vi "Adapt FP.vi"(8 "error in":errorcluster, 11 "ref":refnum<vi>) -> (0 "error out":errorcluster)   [LabVIEW 2009, in "POLARIS Vision utility.lvlib"]
uses:
  POLARIS Vision utility.lvlib
  control position.ctl
  <vilib>/Utility/miscctls.llb/LVPositionTypeDef.ctl
  <vilib>/Utility/miscctls.llb/LVBoundsTypeDef.ctl
  <vilib>/Utility/xml.llb/Write to XML File(string).vi
panel:
  in  "thin":bool
  in  "thick":bool
  in  "wide":bool
  in  "narroq":bool
  in  "bottom":bool
  in  "Top":bool
  in  "Right":bool
  in  "Left":bool
  in  "stop":bool
  in  "Select Element":u16(ring) items=["Numeric", "String", "String 2", "stop", "Path"]
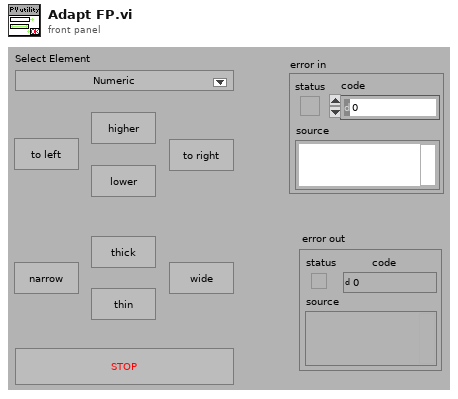
[diagram p1: front panel]
types:
  T1 = typedef "control position.ctl" = cluster{"ControlName":string, "Position":T2, "Size":T3}
  T2 = typedef "LVPositionTypeDef.ctl" = cluster{"Left":i32, "Top":i32}
  T3 = typedef "LVBoundsTypeDef.ctl" = cluster{"Width":u32, "Height":u32}
  T4 = enum32{"invalid app kind", "Development System", "Run Time System", "Student Edition", "Embedded LabVIEW", "Evaluation", "Custom"}
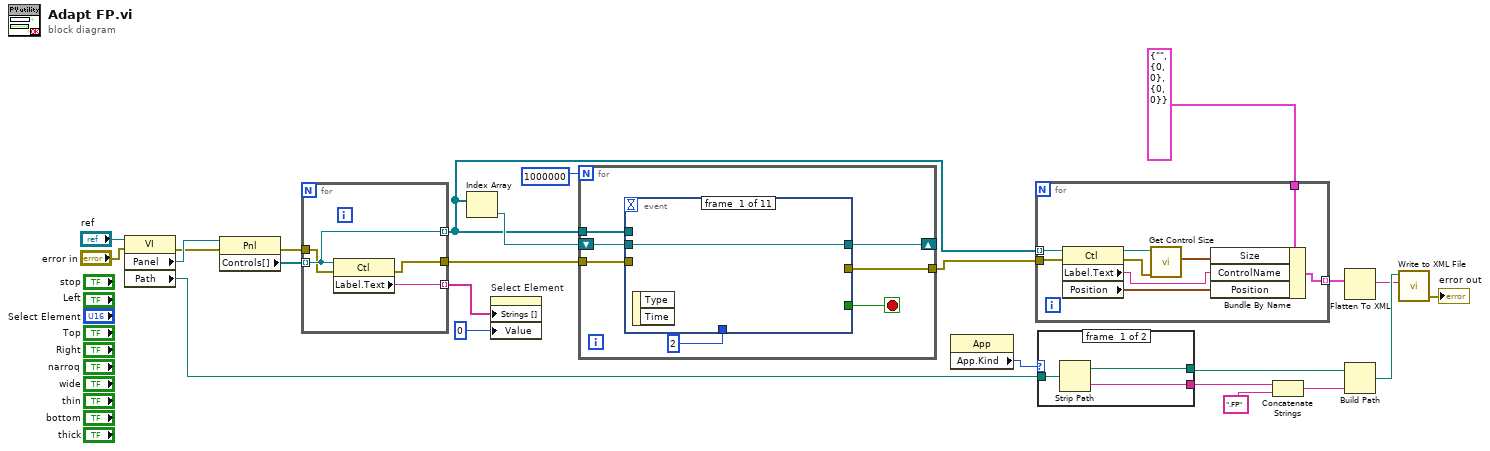
[diagram p0: block diagram]
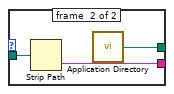
[diagram p2: hidden frame]
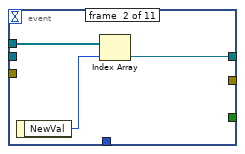
[diagram p3: hidden frame]
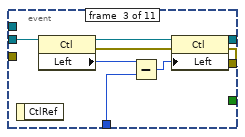
[diagram p4: hidden frame]
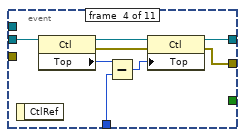
[diagram p5: hidden frame]
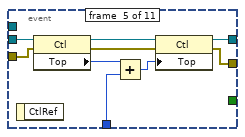
[diagram p6: hidden frame]
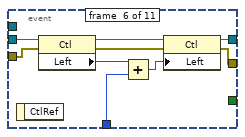
[diagram p7: hidden frame]
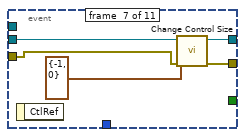
[diagram p8: hidden frame]
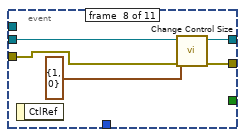
[diagram p9: hidden frame]
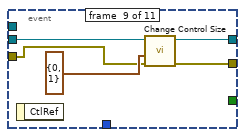
[diagram p10: hidden frame]
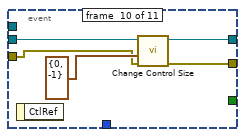
[diagram p11: hidden frame]
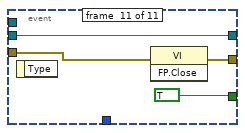
[diagram p12: hidden frame]
diagram:
  n1 = property class="VI"(reference="ref", error in="error in") -> (error out=w22:errorcluster, "Panel"=w23:refnum<vi>, "Path"=w17:path)  [unwired: 1 out]
  n2 = property class="Pnl"(reference=w23, error in=w22) -> (error out=w6:errorcluster, "Controls[]"=w21:refnum<vi>[])  [unwired: 1 out]
  n3 = for {
    tunnel: w21 -> [w27] mode=indexing
    tunnel: [w28] -> w20 mode=indexing
    tunnel: [w27] -> w1 mode=indexing
    tunnel: w6 -> [w26]
    tunnel: [w25] -> w5
    n4 = property class="Ctl"(reference=w27, error in=w26) -> (error out=w25:errorcluster, "Label.Text"=w28:string)  [unwired: 1 out]
  }
  n5 = Index Array(array=w1) -> (element=w19:refnum<vi>)  [unwired: 1 in]
  n6 = property on="Select Element" class="Ring (strict)"("Strings []"=w20, "Value"=u16 0 ("Select Element")) -> ()  [unwired: 2 in, 2 out]
  n7 = for {
    N: 1000000 -> [_]
    tunnel: w1 -> [w35]
    shift-right: [w31] -> _
    shift-left: w19 -> [w34]
    tunnel: [w33] -> w4
    tunnel: w5 -> [w30]
    stop <- w32 stop-if-true
    n8 = event shown="[10] \"stop\": Value Change" {
      selector: _ -> [_ _ _ _ _ _ _ _ _ _ _]
      dyn-events: _ -> [_ _ _ _ _ _ _ _ _ _ _]
      timeout: _ -> [_ _ _ _ _ _ _ _ _ _ _]
      tunnel: w35 -> [_ w39 _ _ _ _ _ _ _ _ _]
      tunnel: [_ _ _ _ _ _ _ _ _ _ TRUE] -> w32
      tunnel: [w36 w38 w43 w51 w60 w69 w78 w83 w88 w93 w96] -> w31
      tunnel: w34 -> [w36 _ w44 w52 w61 w73 w77 w82 w87 w92 w96]
      tunnel: [_ _ w42 w49 w58 w67 w75 w80 w85 w90 w95] -> w33
      tunnel: w30 -> [_ _ _ _ w57 w66 w74 w79 w84 w89 w94]
      tunnel: 2 ("y") -> [_ _ w40 w48 w56 w65 _ _ _ _ _]
      event #0 {
        n9 = event-data() -> ()  [unwired: 1 in, 2 out]
      }
      event #1 {
        n10 = event-data() -> ("NewVal"=w37:u16)  [unwired: 1 in]
        n11 = Index Array(array=w39, index=w37) -> (element=w38:refnum<vi>)
      }
      event #2 {
        n12 = event-data() -> ()  [unwired: 1 in, 1 out]
        n13 = property class="Ctl"(reference=w44) -> (reference out=w45:refnum<vi>, error out=w41:errorcluster, "Left"=w47:i32)  [unwired: 1 in]
        n14 = Subtract(x=w47, y=w40) -> (x-y=w46:i32)
        n15 = property class="Ctl"(reference=w45, error in=w41, "Left"=w46) -> (reference out=w43:refnum<vi>, error out=w42:errorcluster)
      }
      event #3 {
        n16 = event-data() -> ()  [unwired: 1 in, 1 out]
        n17 = property class="Ctl"(reference=w52) -> (reference out=w53:refnum<vi>, error out=w50:errorcluster, "Top"=w55:i32)  [unwired: 1 in]
        n18 = Subtract(x=w55, y=w48) -> (x-y=w54:i32)
        n19 = property class="Ctl"(reference=w53, error in=w50, "Top"=w54) -> (reference out=w51:refnum<vi>, error out=w49:errorcluster)
      }
      event #4 {
        n20 = event-data() -> ()  [unwired: 1 in, 1 out]
        n21 = property class="Ctl"(reference=w61, error in=w57) -> (reference out=w62:refnum<vi>, error out=w59:errorcluster, "Top"=w64:i32)
        n22 = Add(x=w64, y=w56) -> (x+y=w63:i32)
        n23 = property class="Ctl"(reference=w62, error in=w59, "Top"=w63) -> (reference out=w60:refnum<vi>, error out=w58:errorcluster)
      }
      event #5 {
        n24 = event-data() -> ()  [unwired: 1 in, 1 out]
        n25 = property class="Ctl"(reference=w73, error in=w66) -> (reference out=w70:refnum<vi>, error out=w68:errorcluster, "Left"=w72:i32)
        n26 = Add(x=w72, y=w65) -> (x+y=w71:i32)
        n27 = property class="Ctl"(reference=w70, error in=w68, "Left"=w71) -> (reference out=w69:refnum<vi>, error out=w67:errorcluster)
      }
      event #6 {
        n28 = event-data() -> ()  [unwired: 1 in, 1 out]
        n29 = call "Change Control Size.vi"("error in (no error)"=w74, "dSize"=cluster{"Width":i32, "Height":i32} {"Width"=-1, "Height"=0}, "Ctl Refnum"=w77) -> ("error out"=w75:errorcluster, "refnum dub"=w78:refnum<vi>)  [unwired: 6 in, 1 out]
      }
      event #7 {
        n30 = event-data() -> ()  [unwired: 1 in, 1 out]
        n31 = call "Change Control Size.vi"("error in (no error)"=w79, "dSize"=cluster{"Width":i32, "Height":i32} {"Width"=1, "Height"=0}, "Ctl Refnum"=w82) -> ("error out"=w80:errorcluster, "refnum dub"=w83:refnum<vi>)  [unwired: 6 in, 1 out]
      }
      event #8 {
        n32 = event-data() -> ()  [unwired: 1 in, 1 out]
        n33 = call "Change Control Size.vi"("error in (no error)"=w84, "dSize"=cluster{"Width":i32, "Height":i32} {"Width"=0, "Height"=1}, "Ctl Refnum"=w87) -> ("error out"=w85:errorcluster, "refnum dub"=w88:refnum<vi>)  [unwired: 6 in, 1 out]
      }
      event #9 {
        n34 = event-data() -> ()  [unwired: 1 in, 1 out]
        n35 = call "Change Control Size.vi"("error in (no error)"=w89, "dSize"=cluster{"Width":i32, "Height":i32} {"Width"=0, "Height"=-1}, "Ctl Refnum"=w92) -> ("error out"=w90:errorcluster, "refnum dub"=w93:refnum<vi>)  [unwired: 6 in, 1 out]
      }
      event #10 {
        n36 = event-data() -> ()  [unwired: 1 in, 1 out]
        n37 = invoke class="VI" method="FP.Close"(error in=w94) -> (error out=w95:errorcluster)  [unwired: 2 in, 2 out]
      }
    }
  }
  n38 = property class="App"() -> ("App.Kind"=w16:T4)  [unwired: 2 in, 2 out]
  n39 = for {
    tunnel: w1 -> [w106] mode=indexing
    tunnel: [w104] -> w11 mode=indexing
    tunnel: T1 {"ControlName"="", "Position"={"Left"=0, "Top"=0}, "Size"={"Width"=0, "Height"=0}} ("Control Position") -> [w103]
    tunnel: w4 -> [w102]
    n40 = property class="Ctl"(reference=w106, error in=w102) -> (reference out=w105:refnum<vi>, error out=w101:errorcluster, "Label.Text"=w99:string, "Position"=w98:T2)
    n41 = call "Get Control Size.vi"("error in (no error)"=w101, "Ctl Refnum"=w105) -> ("Size"=w100:T3)  [unwired: 6 in, 3 out]
    n42 = Bundle By Name(cluster=w103, "Size"=w100, "ControlName"=w99, "Position"=w98) -> (w104:T1)
  }
  n43 = case shown="\"Development System\", Default" w16 {
    tunnel: w17 -> [w109 w112]
    tunnel: [w108 w111] -> w12
    tunnel: [w107 w110] -> w14
    frame #0 {
      n44 = Strip Path(path=w109) -> (stripped path=w108:path, name=w107:string)
    }
    frame #1 {
      n45 = Strip Path(path=w112) -> (name=w110:string)  [unwired: 1 out]
      n46 = call <vilib>:"Application Directory.vi"() -> ("Application Directory"=w111:path)
    }
  }
  n47 = Concatenate Strings(w14, ".FP" ("string")) -> (w13:string)
  n48 = Flatten To XML(anything=w11) -> (xml string=w9:string)
  n49 = Build Path(base path=w12, name or relative path=w13) -> (appended path=w10:path)
  n50 = call-poly <vilib>:"Write to XML File.vi"("XML Input"=w9, "XML File Path"=w10) -> ("error out"=→"error out":errorcluster)  [unwired: 7 in, 2 out]
